vi "Run Bookmark Manager Unit Tests.vi"(8 "Error In":errorcluster) -> (0 "Error Out":errorcluster)   [LabVIEW 2018, in "Scripts.lvlib"]
uses:
  Scripts.lvlib
  <vilib>/addons/_JKI Toolkits/Caraya/classes/Test/Test.lvclass
  tests/Bookmark Manager/Unit/Unit.lvlib
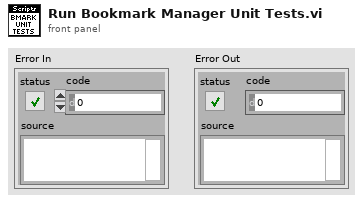
[diagram p1: front panel]
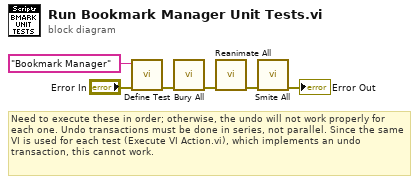
[diagram p0: block diagram]
diagram:
  # "Need to execute these in order; otherwise, the undo will not work properly for each one. Undo transactions must be done in series, not parallel. Since the same VI is used for each test (Execute VI Action.vi), which implements an undo transaction, this cannot work."
  n1 = call <vilib>:"Define Test.vi"("error in (no error)"="Error In", "Label (VI Title)"="Bookmark Manager") -> ("error out"=w2:errorcluster)  [unwired: 9 in]
  n2 = call "Bury All.vi"("Error In"=w2) -> ("Error Out"=w4:errorcluster)  [unwired: 10 in]
  n3 = call "Reanimate All.vi"("Error In"=w4) -> ("Error Out"=w3:errorcluster)  [unwired: 10 in]
  n4 = call "Smite All.vi"("Error In"=w3) -> ("Error Out"=→"Error Out":errorcluster)  [unwired: 10 in]
